vi "test_read-nmea-data2.vi"() -> ()   [LabVIEW 2019] (continued)
,57.96,250720,,,A,V*3D\n\t\n15:12:59.26\tF9P\t$GNVTG,57.96,T,,M,2.140,N,3.964,K,A*11\n\t\n15:12:59.28\tF9P\t$GNGGA,061301.00,3723.55169,N,12656.96549,E,1,12,0.94,42.1,M,18.5,M,,*78\n\t\n15:12:59.30\tF9P\t$GNGSA,A,3,12,06,19,05,17,09,04,02,,,,,1.64,0.94,1.34,1*08\n\t\n15:12:59.32\tF9P\t$GNGSA,A,3,85,70,71,84,,,,,,,,,1.64,0.94,1.34,2*0A\n\t\n15:12:59.34\tF9P\t$GNGSA,A,3,36,19,11,04,09,12,,,,,,,1.64,0.94,1.34,3*08\n\t\n15:12:59.36\tF9P\t$GNGSA,A,3,14,11,33,,,,,,,,,,1.64,0.94,1.34,4*09\n\t\n15:12:59.38\tF9P\t$GPGSV,3,1,09,02,55,319,21,04,18,043,25,05,37,247,27,06,64,049,31,1*66\n\t\n15:12:59.40\tF9P\t$GPGSV,3,2,09,09,45,074,34,12,23,276,25,17,33,154,30,19,52,157,31,1*6D\n\t\n15:12:59.42\tF9P\t$GPGSV,3,3,09,25,12,306,21,1*5F\n\t\n15:12:59.44\tF9P\t$GPGSV,3,1,09,02,55,319,,04,18,043,21,05,37,247,21,06,64,049,24,6*64\n\t\n15:12:59.46\tF9P\t$GPGSV,3,2,09,09,45,074,28,12,23,276,16,17,33,154,19,19,52,157,,6*6E\n\t\n15:12:59.48\tF9P\t$GPGSV,3,3,09,25,12,306,,6*5B\n\t\n15:12:59.50\tF9P\t$GLGSV,2,1,08,69,11,031,25,70,70,038,28,71,53,206,37,72,05,210,23,1*7A\n\t\n15:12:59.52\tF9P\t$GLGSV,2,2,08,77,01,326,,84,20,122,12,85,70,067,35,86,37,330,,1*7D\n\t\n15:12:59.54\tF9P\t$GLGSV,2,1,08,69,11,031,14,70,70,038,,71,53,206,26,72,05,210,,3*71\n\t\n15:12:59.56\tF9P\t$GLGSV,2,2,08,77,01,326,,84,20,122,19,85,70,067,29,86,37,330,,3*79\n\t\n15:12:59.58\tF9P\t$GAGSV,2,1,08,02,08,297,08,04,66,116,27,09,32,193,34,11,72,359,26,7*7B\n\t\n15:12:59.60\tF9P\t$GAGSV,2,2,08,12,40,103,33,19,26,045,22,25,09,249,,36,26,308,16,7*7F\n\t\n15:12:59.62\tF9P\t$GAGSV,2,1,08,02,08,297,,04,66,116,,09,32,193,32,11,72,359,,2*71\n\t\n15:12:59.64\tF9P\t$GAGSV,2,2,08,12,40,103,,19,26,045,,25,09,249,,36,26,308,,2*7D\n\t\n15:12:59.66\tF9P\t$GBGSV,1,1,04,11,49,132,24,14,87,114,27,28,,,20,33,61,220,35,1*4B\n\t\n15:12:59.68\tF9P\t$GBGSV,1,1,03,11,49,132,,14,87,114,27,33,61,220,,3*46\n\t\n15:12:59.70\tF9P\t$GNGLL,3723.55169,N,12656.96549,E,061301.00,A,A*78\n\t\n15:12:59.72\tF9P\t\t\n15:12:59.74\tF9P\t\t\n15:12:59.76\tF9P\t\t\n15:12:59.78\tF9P\t\t\n15:12:59.80\tF9P\t\t\n15:12:59.82\tF9P\t\t\n15:12:59.84\tF9P\t\t\n15:12:59.86\tF9P\t\t\n15:12:59.88\tF9P\t\t\n15:12:59.90\tF9P\t\t\n15:12:59.92\tF9P\t\t\n15:12:59.94\tF9P\t\t\n15:12:59.96\tF9P\t\t\n15:12:59.98\tF9P\t\t\n15:13:00.00\tF9P\t\t\n15:13:00.02\tF9P\t\t\n15:13:00.04\tF9P\t\t\n15:13:00.06\tF9P\t\t\n15:13:00.08\tF9P\t\t\n15:13:00.10\tF9P\t\t\n15:13:00.12\tF9P\t\t\n15:13:00.14\tF9P\t\t\n15:13:00.16\tF9P\t\t\n15:13:00.18\tF9P\t\t\n15:13:00.20\tF9P\t\t\n15:13:00.22\tF9P\t\t\n15:13:00.24\tF9P\t$GNRMC,061302.00,A,3723.55217,N,12656.96618,E,2.079,53.79,250720,,,A,V*3D\n\t\n15:13:00.26\tF9P\t$GNVTG,53.79,T,,M,2.079,N,3.851,K,A*18\n\t\n15:13:00.28\tF9P\t$GNGGA,061302.00,3723.55217,N,12656.96618,E,1,12,0.93,42.2,M,18.5,M,,*72\n\t\n15:13:00.30\tF9P\t$GNGSA,A,3,12,06,19,05,17,09,04,02,,,,,1.63,0.93,1.34,1*08\n\t\n15:13:00.32\tF9P\t$GNGSA,A,3,85,70,71,84,,,,,,,,,1.63,0.93,1.34,2*0A\n\t\n15:13:00.34\tF9P\t$GNGSA,A,3,36,19,11,04,09,12,,,,,,,1.63,0.93,1.34,3*08\n\t\n15:13:00.36\tF9P\t$GNGSA,A,3,14,11,33,,,,,,,,,,1.63,0.93,1.34,4*09\n\t\n15:13:00.38\tF9P\t$GPGSV,3,1,09,02,55,319,21,04,18,043,24,05,37,247,26,06,64,049,25,1*63\n\t\n15:13:00.40\tF9P\t$GPGSV,3,2,09,09,45,074,29,12,23,276,,17,33,154,33,19,52,157,29,1*6C\n\t\n15:13:00.42\tF9P\t$GPGSV,3,3,09,25,12,306,21,1*5F\n\t\n15:13:00.44\tF9P\t$GPGSV,3,1,09,02,55,319,,04,18,043,22,05,37,247,20,06,64,049,26,6*64\n\t\n15:13:00.46\tF9P\t$GPGSV,3,2,09,09,45,074,28,12,23,276,13,17,33,154,19,19,52,157,,6*6B\n\t\n15:13:00.48\tF9P\t$GPGSV,3,3,09,25,12,306,,6*5B\n\t\n15:13:00.50\tF9P\t$GLGSV,2,1,08,69,11,031,23,70,70,038,30,71,53,206,38,72,05,210,23,1*7A\n\t\n15:13:00.52\tF9P\t$GLGSV,2,2,08,77,01,326,,84,20,122,13,85,70,067,31,86,37,330,,1*78\n\t\n15:13:00.54\tF9P\t$GLGSV,2,1,08,69,11,031,15,70,70,038,,71,53,206,25,72,05,210,,3*73\n\t\n15:13:00.56\tF9P\t$GLGSV,2,2,08,77,01,326,,84,20,122,18,85,70,067,23,86,37,330,,3*72\n\t\n15:13:00.58\tF9P\t$GAGSV,2,1,08,02,08,297,12,04,66,116,28,09,32,193,33,11,72,359,31,7*7E\n\t\n15:13:00.60\tF9P\t$GAGSV,2,2,08,12,40,103,32,19,26,045,24,25,09,249,,36,26,308,15,7*7B\n\t\n15:13:00.62\tF9P\t$GAGSV,2,1,08,02,08,297,,04,66,116,,09,32,193,,11,72,359,,2*70\n\t\n15:13:00.64\tF9P\t$GAGSV,2,2,08,12,40,103,,19,26,045,,25,09,249,,36,26,308,,2*7D\n\t\n15:13:00.66\tF9P\t$GBGSV,1,1,04,11,49,132,30,14,87,114,28,28,,,21,33,61,220,27,1*43\n\t\n15:13:00.68\tF9P\t$GBGSV,1,1,03,11,49,132,,14,87,114,,33,61,220,,3*43\n\t\n15:13:00.70\tF9P\t$GNGLL,3723.55217,N,12656.96618,E,061302.00,A,A*76\n\t\n15:13:00.72\tF9P\t\t\n15:13:00.74\tF9P\t\t\n15:13:00.76\tF9P\t\t\n15:13:00.78\tF9P\t\t\n15:13:00.80\tF9P\t\t\n15:13:00.82\tF9P\t\t\n15:13:00.84\tF9P\t\t\n15:13:00.86\tF9P\t\t\n15:13:00.88\tF9P\t\t\n15:13:00.90\tF9P\t\t\n15:13:00.92\tF9P\t\t\n15:13:00.94\tF9P\t\t\n15:13:00.96\tF9P\t\t\n15:13:00.98\tF9P\t\t\n15:13:01.00\tF9P\t\t\n15:13:01.02\tF9P\t\t\n15:13:01.04\tF9P\t\t\n15:13:01.06\tF9P\t\t\n15:13:01.08\tF9P\t\t\n15:13:01.10\tF9P\t\t\n15:13:01.12\tF9P\t\t\n15:13:01.14\tF9P\t\t\n15:13:01.16\tF9P\t\t\n15:13:01.18\tF9P\t\t\n15:13:01.20\tF9P\t\t\n15:13:01.22\tF9P\t\t\n15:13:01.24\tF9P\t$GNRMC,061303.00,A,3723.55265,N,12656.96684,E,2.088,52.28,250720,,,A,V*37\n\t\n15:13:01.26\tF9P\t$GNVTG,52.28,T,,M,2.088,N,3.867,K,A*16\n\t\n15:13:01.28\tF9P\t$GNGGA,061303.00,3723.55265,N,12656.96684,E,1,12,0.93,42.2,M,18.5,M,,*73\n\t\n15:13:01.30\tF9P\t$GNGSA,A,3,06,19,05,17,09,04,02,,,,,,1.63,0.93,1.34,1*0B\n\t\n15:13:01.32\tF9P\t$GNGSA,A,3,85,70,71,84,,,,,,,,,1.63,0.93,1.34,2*0A\n\t\n15:13:01.34\tF9P\t$GNGSA,A,3,36,19,11,04,09,12,,,,,,,1.63,0.93,1.34,3*08\n\t\n15:13:01.36\tF9P\t$GNGSA,A,3,14,11,33,,,,,,,,,,1.63,0.93,1.34,4*09\n\t\n15:13:01.38\tF9P\t$GPGSV,3,1,09,02,55,319,21,04,18,043,25,05,37,247,35,06,64,049,34,1*60\n\t\n15:13:01.40\tF9P\t$GPGSV,3,2,09,09,45,074,33,12,23,276,23,17,33,154,29,19,52,157,34,1*61\n\t\n15:13:01.42\tF9P\t$GPGSV,3,3,09,25,12,306,21,1*5F\n\t\n15:13:01.44\tF9P\t$GPGSV,3,1,09,02,55,319,,04,18,043,21,05,37,247,21,06,64,049,25,6*65\n\t\n15:13:01.46\tF9P\t$GPGSV,3,2,09,09,45,074,26,12,23,276,,17,33,154,20,19,52,157,,6*6D\n\t\n15:13:01.48\tF9P\t$GPGSV,3,3,09,25,12,306,,6*5B\n\t\n15:13:01.50\tF9P\t$GLGSV,2,1,08,69,11,031,23,70,70,038,30,71,53,206,39,72,05,210,23,1*7B\n\t\n15:13:01.52\tF9P\t$GLGSV,2,2,08,77,01,326,,84,20,122,10,85,70,067,29,86,37,330,,1*72\n\t\n15:13:01.54\tF9P\t$GLGSV,2,1,08,69,11,031,17,70,70,038,,71,53,206,25,72,05,210,,3*71\n\t\n15:13:01.56\tF9P\t$GLGSV,2,2,08,77,01,326,,84,20,122,20,85,70,067,22,86,37,330,,3*78\n\t\n15:13:01.58\tF9P\t$GAGSV,2,1,08,02,08,297,12,04,66,116,28,09,32,193,34,11,72,359,31,7*79\n\t\n15:13:01.60\tF9P\t$GAGSV,2,2,08,12,40,103,28,19,26,045,24,25,09,249,,36,26,308,15,7*70\n\t\n15:13:01.62\tF9P\t$GAGSV,2,1,08,02,08,297,,04,66,116,,09,32,193,,11,72,359,,2*70\n\t\n15:13:01.64\tF9P\t$GAGSV,2,2,08,12,40,103,,19,26,045,,25,09,249,,36,26,308,,2*7D\n\t\n15:13:01.66\tF9P\t$GBGSV,1,1,04,11,49,132,29,14,87,114,32,28,,,20,33,61,220,32,1*45\n\t\n15:13:01.68\tF9P\t$GBGSV,1,1,03,11,49,132,,14,87,114,27,33,61,220,,3*46\n\t\n15:13:01.70\tF9P\t$GNGLL,3723.55265,N,12656.96684,E,061303.00,A,A*77\n\t\n15:13:01.72\tF9P\t\t\n15:13:01.74\tF9P\t\t\n15:13:01.76\tF9P\t\t\n15:13:01.78\tF9P\t\t\n15:13:01.80\tF9P\t\t\n15:13:01.82\tF9P\t\t\n15:13:01.84\tF9P\t\t\n15:13:01.86\tF9P\t\t\n15:13:01.88\tF9P\t\t\n15:13:01.90\tF9P\t\t\n15:13:01.92\tF9P\t\t\n15:13:01.94\tF9P\t\t\n15:13:01.96\tF9P\t\t\n15:13:01.98\tF9P\t\t\n15:13:02.00\tF9P\t\t\n15:13:02.02\tF9P\t\t\n15:13:02.04\tF9P\t\t\n15:13:02.06\tF9P\t\t\n15:13:02.08\tF9P\t\t\n15:13:02.10\tF9P\t\t\n15:13:02.12\tF9P\t\t\n15:13:02.14\tF9P\t\t\n15:13:02.16\tF9P\t\t\n15:13:02.18\tF9P\t\t\n15:13:02.20\tF9P\t\t\n15:13:02.22\tF9P\t\t\n15:13:02.24\tF9P\t$GNRMC,061304.00,A,3723.55321,N,12656.96735,E,1.731,50.68,250720,,,A,V*3A\n\t\n15:13:02.26\tF9P\t$GNVTG,50.68,T,,M,1.731,N,3.206,K,A*1B\n\t\n15:13:02.28\tF9P\t$GNGGA,061304.00,3723.55321,N,12656.96735,E,1,12,0.93,42.3,M,18.5,M,,*7F\n\t\n15:13:02.30\tF9P\t$GNGSA,A,3,06,19,05,17,09,04,02,,,,,,1.63,0.93,1.34,1*0B\n\t\n15:13:02.32\tF9P\t$GNGSA,A,3,85,70,71,84,,,,,,,,,1.63,0.93,1.34,2*0A\n\t\n15:13:02.34\tF9P\t$GNGSA,A,3,36,19,11,04,09,12,,,,,,,1.63,0.93,1.34,3*08\n\t\n15:13:02.36\tF9P\t$GNGSA,A,3,14,11,33,,,,,,,,,,1.63,0.93,1.34,4*09\n\t\n15:13:02.38\tF9P\t$GPGSV,3,1,09,02,55,319,22,04,18,043,26,05,37,247,30,06,64,049,25,1*65\n\t\n15:13:02.40\tF9P\t$GPGSV,3,2,09,09,45,074,31,12,23,276,23,17,33,154,28,19,52,157,30,1*66\n\t\n15:13:02.42\tF9P\t$GPGSV,3,3,09,25,12,306,20,1*5E\n\t\n15:13:02.44\tF9P\t$GPGSV,3,1,09,02,55,319,,04,18,043,19,05,37,247,22,06,64,049,25,6*6D\n\t\n15:13:02.46\tF9P\t$GPGSV,3,2,09,09,45,074,28,12,23,276,,17,33,154,20,19,52,157,,6*63\n\t\n15:13:02.48\tF9P\t$GPGSV,3,3,09,25,12,306,,6*5B\n\t\n15:13:02.50\tF9P\t$GLGSV,2,1,08,69,11,031,23,70,70,038,31,71,53,206,42,72,05,210,23,1*76\n\t\n15:13:02.52\tF9P\t$GLGSV,2,2,08,77,01,326,,84,20,122,15,85,70,067,34,86,37,330,,1*7B\n\t\n15:13:02.54\tF9P\t$GLGSV,2,1,08,69,11,031,16,70,70,038,,71,53,206,25,72,05,210,,3*70\n\t\n15:13:02.56\tF9P\t$GLGSV,2,2,08,77,01,326,,84,20,122,20,85,70,067,21,86,37,330,,3*7B\n\t\n15:13:02.58\tF9P\t$GAGSV,2,1,08,02,08,297,09,04,66,116,28,09,32,193,37,11,72,359,35,7*74\n\t\n15:13:02.60\tF9P\t$GAGSV,2,2,08,12,40,103,28,19,26,045,24,25,09,249,,36,26,308,16,7*73\n\t\n15:13:02.62\tF9P\t$GAGSV,2,1,08,02,08,297,,04,66,116,,09,32,193,,11,72,359,,2*70\n\t\n15:13:02.64\tF9P\t$GAGSV,2,2,08,12,40,103,,19,26,045,,25,09,249,,36,26,308,,2*7D\n\t\n15:13:02.66\tF9P\t$GBGSV,1,1,04,11,49,132,28,14,87,114,28,28,,,20,33,61,220,30,1*4D\n\t\n15:13:02.68\tF9P\t$GBGSV,1,1,03,11,49,132,,14,87,114,27,33,61,220,,3*46\n\t\n15:13:02.70\tF9P\t$GNGLL,3723.55321,N,12656.96735,E,061304.00,A,A*7A\n\t\n15:13:02.72\tF9P\t\t\n15:13:02.74\tF9P\t\t\n15:13:02.76\tF9P\t\t\n15:13:02.78\tF9P\t\t\n15:13:02.80\tF9P\t\t\n15:13:02.82\tF9P\t\t\n15:13:02.84\tF9P\t\t\n15:13:02.86\tF9P\t\t\n15:13:02.88\tF9P\t\t\n15:13:02.90\tF9P\t\t\n15:13:02.92\tF9P\t\t\n15:13:02.94\tF9P\t\t\n15:13:02.96\tF9P\t\t\n15:13:02.98\tF9P\t\t\n15:13:03.00\tF9P\t\t\n15:13:03.02\tF9P\t\t\n15:13:03.04\tF9P\t\t\n15:13:03.06\tF9P\t\t\n15:13:03.08\tF9P\t\t\n15:13:03.10\tF9P\t\t\n15:13:03.12\tF9P\t\t\n15:13:03.14\tF9P\t\t\n15:13:03.16\tF9P\t\t\n15:13:03.18\tF9P\t\t\n15:13:03.20\tF9P\t\t\n15:13:03.22\tF9P\t\t\n15:13:03.24\tF9P\t$GNRMC,061305.00,A,3723.55365,N,12656.96800,E,2.177,53.20,250720,,,A,V*3A\n\t\n15:13:03.26\tF9P\t$GNVTG,53.20,T,,M,2.177,N,4.032,K,A*11\n\t\n15:13:03.28\tF9P\t$GNGGA,061305.00,3723.55365,N,12656.96800,E,1,12,0.93,42.1,M,18.5,M,,*75\n\t\n15:13:03.30\tF9P\t$GNGSA,A,3,12,06,19,05,17,09,04,02,,,,,1.63,0.93,1.34,1*08\n\t\n15:13:03.32\tF9P\t$GNGSA,A,3,85,70,71,84,,,,,,,,,1.63,0.93,1.34,2*0A\n\t\n15:13:03.34\tF9P\t$GNGSA,A,3,36,19,11,04,09,12,,,,,,,1.63,0.93,1.34,3*08\n\t\n15:13:03.36\tF9P\t$GNGSA,A,3,14,11,33,,,,,,,,,,1.63,0.93,1.34,4*09\n\t\n15:13:03.38\tF9P\t$GPGSV,3,1,09,02,55,319,22,04,18,043,25,05,37,247,29,06,64,049,25,1*6E\n\t\n15:13:03.40\tF9P\t$GPGSV,3,2,09,09,45,074,28,12,23,276,22,17,33,154,29,19,52,157,30,1*6E\n\t\n15:13:03.42\tF9P\t$GPGSV,3,3,09,25,12,306,20,1*5E\n\t\n15:13:03.44\tF9P\t$GPGSV,3,1,09,02,55,319,,04,18,043,17,05,37,247,22,06,64,049,26,6*60\n\t\n15:13:03.46\tF9P\t$GPGSV,3,2,09,09,45,074,27,12,23,276,,17,33,154,20,19,52,157,,6*6C\n\t\n15:13:03.48\tF9P\t$GPGSV,3,3,09,25,12,306,,6*5B\n\t\n15:13:03.50\tF9P\t$GLGSV,2,1,08,69,11,031,30,70,70,038,26,71,53,206,42,72,05,210,23,1*72\n\t\n15:13:03.52\tF9P\t$GLGSV,2,2,08,77,01,326,,84,20,122,11,85,70,067,38,86,37,330,,1*73\n\t\n15:13:03.54\tF9P\t$GLGSV,2,1,08,69,11,031,18,70,70,038,,71,53,206,23,72,05,210,,3*78\n\t\n15:13:03.56\tF9P\t$GLGSV,2,2,08,77,01,326,,84,20,122,19,85,70,067,22,86,37,330,,3*72\n\t\n15:13:03.58\tF9P\t$GAGSV,2,1,08,02,08,297,08,04,66,116,28,09,32,193,36,11,72,359,29,7*79\n\t\n15:13:03.60\tF9P\t$GAGSV,2,2,08,12,40,103,28,19,26,045,25,25,09,249,,36,26,308,15,7*71\n\t\n15:13:03.62\tF9P\t$GAGSV,2,1,08,02,08,297,,04,66,116,,09,32,193,,11,72,359,,2*70\n\t\n15:13:03.64\tF9P\t$GAGSV,2,2,08,12,40,103,,19,26,045,,25,09,249,,36,26,308,,2*7D\n\t\n15:13:03.66\tF9P\t$GBGSV,1,1,04,11,49,132,29,14,87,114,29,28,,,19,33,61,220,33,1*44\n\t\n15:13:03.68\tF9P\t$GBGSV,1,1,03,11,49,132,,14,87,114,27,33,61,220,,3*46\n\t\n15:13:03.70\tF9P\t$GNGLL,3723.55365,N,12656.96800,E,061305.00,A,A*72\n\t\n15:13:03.72\tF9P\t\t\n15:13:03.74\tF9P\t\t\n15:13:03.76\tF9P\t\t\n15:13:03.78\tF9P\t\t\n15:13:03.80\tF9P\t\t\n15:13:03.82\tF9P\t\t\n15:13:03.84\tF9P\t\t\n15:13:03.86\tF9P\t\t\n15:13:03.88\tF9P\t\t\n15:13:03.90\tF9P\t\t\n15:13:03.92\tF9P\t\t\n15:13:03.94\tF9P\t\t\n15:13:03.96\tF9P\t\t\n15:13:03.98\tF9P\t\t\n15:13:04.00\tF9P\t\t\n15:13:04.02\tF9P\t\t\n15:13:04.04\tF9P\t\t\n15:13:04.06\tF9P\t\t\n15:13:04.08\tF9P\t\t\n15:13:04.10\tF9P\t\t\n15:13:04.12\tF9P\t\t\n15:13:04.14\tF9P\t\t\n15:13:04.16\tF9P\t\t\n15:13:04.18\tF9P\t\t\n15:13:04.20\tF9P\t\t\n15:13:04.22\tF9P\t\t\n15:13:04.24\tF9P\t$GNRMC,061306.00,A,3723.55373,N,12656.96887,E,2.176,59.83,250720,,,A,V*33\n\t\n15:13:04.26\tF9P\t$GNVTG,59.83,T,,M,2.176,N,4.029,K,A*19\n\t\n15:13:04.28\tF9P\t$GNGGA,061306.00,3723.55373,N,12656.96887,E,1,12,0.93,43.8,M,18.5,M,,*76\n\t\n15:13:04.30\tF9P\t$GNGSA,A,3,12,06,19,05,17,09,04,02,,,,,1.63,0.93,1.34,1*08\n\t\n15:13:04.32\tF9P\t$GNGSA,A,3,85,70,71,84,,,,,,,,,1.63,0.93,1.34,2*0A\n\t\n15:13:04.34\tF9P\t$GNGSA,A,3,36,19,11,04,09,12,,,,,,,1.63,0.93,1.34,3*08\n\t\n15:13:04.36\tF9P\t$GNGSA,A,3,14,11,33,,,,,,,,,,1.63,0.93,1.34,4*09\n\t\n15:13:04.38\tF9P\t$GPGSV,3,1,09,02,55,319,22,04,18,043,25,05,37,247,33,06,64,049,31,1*60\n\t\n15:13:04.40\tF9P\t$GPGSV,3,2,09,09,45,074,29,12,23,276,21,17,33,154,29,19,52,157,30,1*6C\n\t\n15:13:04.42\tF9P\t$GPGSV,3,3,09,25,12,306,20,1*5E\n\t\n15:13:04.44\tF9P\t$GPGSV,3,1,09,02,55,319,,04,18,043,17,05,37,247,21,06,64,049,24,6*61\n\t\n15:13:04.46\tF9P\t$GPGSV,3,2,09,09,45,074,28,12,23,276,,17,33,154,20,19,52,157,,6*63\n\t\n15:13:04.48\tF9P\t$GPGSV,3,3,09,25,12,306,,6*5B\n\t\n15:13:04.50\tF9P\t$GLGSV,2,1,08,69,11,031,25,70,70,038,26,71,53,206,41,72,05,210,21,1*77\n\t\n15:13:04.52\tF9P\t$GLGSV,2,2,08,77,01,325,,84,20,122,12,85,70,067,32,86,37,330,,1*79\n\t\n15:13:04.54\tF9P\t$GLGSV,2,1,08,69,11,031,16,70,70,038,,71,53,206,24,72,05,210,,3*71\n\t\n15:13:04.56\tF9P\t$GLGSV,2,2,08,77,01,325,,84,20,122,19,85,70,067,23,86,37,330,,3*70\n\t\n15:13:04.58\tF9P\t$GAGSV,2,1,08,02,08,297,10,04,66,116,28,09,32,193,38,11,72,359,32,7*74\n\t\n15:13:04.60\tF9P\t$GAGSV,2,2,08,12,40,103,29,19,26,045,25,25,09,249,,36,26,308,14,7*71\n\t\n15:13:04.62\tF9P\t$GAGSV,2,1,08,02,08,297,,04,66,116,,09,32,193,,11,72,359,,2*70\n\t\n15:13:04.64\tF9P\t$GAGSV,2,2,08,12,40,103,,19,26,045,,25,09,249,,36,26,308,,2*7D\n\t\n15:13:04.66\tF9P\t$GBGSV,1,1,04,11,49,132,30,14,87,114,22,28,,,19,33,61,220,32,1*46\n\t\n15:13:04.68\tF9P\t$GBGSV,1,1,03,11,49,132,,14,87,114,26,33,61,220,,3*47\n\t\n15:13:04.70\tF9P\t$GNGLL,3723.55373,N,12656.96887,E,061306.00,A,A*79\n\t\n15:13:04.72\tF9P\t\t\n15:13:04.74\tF9P\t\t\n15:13:04.76\tF9P\t\t\n15:13:04.78\tF9P\t\t\n15:13:04.80\tF9P\t\t\n15:13:04.82\tF9P\t\t\n15:13:04.84\tF9P\t\t\n15:13:04.86\tF9P\t\t\n15:13:04.88\tF9P\t\t\n15:13:04.90\tF9P\t\t\n15:13:04.92\tF9P\t\t\n15:13:04.94\tF9P\t\t\n15:13:04.96\tF9P\t\t\n15:13:04.98\tF9P\t\t\n15:13:05.00\tF9P\t\t\n15:13:05.02\tF9P\t\t\n15:13:05.04\tF9P\t\t\n15:13:05.06\tF9P\t\t\n15:13:05.08\tF9P\t\t\n15:13:05.10\tF9P\t\t\n15:13:05.12\tF9P\t\t\n15:13:05.14\tF9P\t\t\n15:13:05.16\tF9P\t\t\n15:13:05.18\tF9P\t\t\n15:13:05.20\tF9P\t\t\n15:13:05.22\tF9P\t\t\n15:13:05.24\tF9P\t$GNRMC,061307.00,A,3723.55392,N,12656.96968,E,2.056,68.99,250720,,,A,V*37\n\t\n15:13:05.26\tF9P\t$GNVTG,68.99,T,,M,2.056,N,3.808,K,A*1F\n\t\n15:13:05.28\tF9P\t$GNGGA,061307.00,3723.55392,N,12656.96968,E,1,12,0.93,43.6,M,18.5,M,,*76\n\t\n15:13:05.30\tF9P\t$GNGSA,A,3,12,06,19,05,17,09,04,02,,,,,1.63,0.93,1.34,1*08\n\t\n15:13:05.32\tF9P\t$GNGSA,A,3,85,70,71,84,,,,,,,,,1.63,0.93,1.34,2*0A\n\t\n15:13:05.34\tF9P\t$GNGSA,A,3,36,19,11,04,09,12,,,,,,,1.63,0.93,1.34,3*08\n\t\n15:13:05.36\tF9P\t$GNGSA,A,3,14,11,33,,,,,,,,,,1.63,0.93,1.34,4*09\n\t\n15:13:05.38\tF9P\t$GPGSV,3,1,09,02,55,319,22,04,18,043,25,05,37,247,35,06,64,049,36,1*61\n\t\n15:13:05.40\tF9P\t$GPGSV,3,2,09,09,45,074,29,12,23,276,22,17,33,154,30,19,52,157,34,1*63\n\t\n15:13:05.42\tF9P\t$GPGSV,3,3,09,25,12,306,20,1*5E\n\t\n15:13:05.44\tF9P\t$GPGSV,3,1,09,02,55,319,,04,18,043,17,05,37,247,20,06,64,049,25,6*61\n\t\n15:13:05.46\tF9P\t$GPGSV,3,2,09,09,45,074,28,12,23,276,,17,33,154,22,19,52,157,,6*61\n\t\n15:13:05.48\tF9P\t$GPGSV,3,3,09,25,12,306,,6*5B\n\t\n15:13:05.50\tF9P\t$GLGSV,2,1,08,69,11,031,25,70,70,038,26,71,53,206,35,72,05,210,20,1*75\n\t\n15:13:05.52\tF9P\t$GLGSV,2,2,08,77,01,325,,84,20,122,13,85,70,067,29,86,37,330,,1*72\n\t\n15:13:05.54\tF9P\t$GLGSV,2,1,08,69,11,031,18,70,70,038,,71,53,206,31,72,05,210,,3*7B\n\t\n15:13:05.56\tF9P\t$GLGSV,2,2,08,77,01,325,,84,20,122,19,85,70,067,25,86,37,330,,3*76\n\t\n15:13:05.58\tF9P\t$GAGSV,2,1,08,02,08,297,12,04,66,116,33,09,32,193,33,11,72,359,27,7*73\n\t\n15:13:05.60\tF9P\t$GAGSV,2,2,08,12,40,103,30,19,26,045,22,25,09,249,,36,26,308,13,7*79\n\t\n15:13:05.62\tF9P\t$GAGSV,2,1,08,02,08,297,,04,66,116,,09,32,193,,11,72,359,,2*70\n\t\n15:13:05.64\tF9P\t$GAGSV,2,2,08,12,40,103,,19,26,045,,25,09,249,,36,26,308,,2*7D\n\t\n15:13:05.66\tF9P\t$GBGSV,1,1,04,11,49,132,33,14,87,114,29,28,,,20,33,61,220,34,1*42\n\t\n15:13:05.68\tF9P\t$GBGSV,1,1,03,11,49,132,,14,87,114,,33,61,220,,3*43\n\t\n15:13:05.70\tF9P\t$GNGLL,3723.55392,N,12656.96968,E,061307.00,A,A*77\n\t\n15:13:05.72\tF9P\t\t\n15:13:05.74\tF9P\t\t\n15:13:05.76\tF9P\t\t\n15:13:05.78\tF9P\t\t\n15:13:05.80\tF9P\t\t\n15:13:05.82\tF9P\t\t\n15:13:05.84\tF9P\t\t\n15:13:05.86\tF9P\t\t\n15:13:05.88\tF9P\t\t\n15:13:05.90\tF9P\t\t\n15:13:05.92\tF9P\t\t\n15:13:05.94\tF9P\t\t\n15:13:05.96\tF9P\t\t\n15:13:05.98\tF9P\t\t\n15:13:06.00\tF9P\t\t\n15:13:06.02\tF9P\t\t\n15:13:06.04\tF9P\t\t\n15:13:06.06\tF9P\t\t\n15:13:06.08\tF9P\t\t\n15:13:06.10\tF9P\t\t\n15:13:06.12\tF9P\t\t\n15:13:06.14\tF9P\t\t\n15:13:06.16\tF9P\t\t\n15:13:06.18\tF9P\t\t\n15:13:06.20\tF9P\t\t\n15:13:06.22\tF9P\t\t\n15:13:06.24\tF9P\t$GNRMC,061308.00,A,3723.55442,N,12656.97048,E,2.371,69.27,250720,,,A,V*3A\n\t\n15:13:06.26\tF9P\t$GNVTG,69.27,T,,M,2.371,N,4.391,K,A*11\n\t\n15:13:06.28\tF9P\t$GNGGA,061308.00,3723.55442,N,12656.97048,E,1,12,0.94,42.4,M,18.5,M,,*7D\n\t\n15:13:06.30\tF9P\t$GNGSA,A,3,12,06,19,05,17,09,04,02,,,,,1.65,0.94,1.35,1*08\n\t\n15:13:06.32\tF9P\t$GNGSA,A,3,85,71,84,,,,,,,,,,1.65,0.94,1.35,2*0D\n\t\n15:13:06.34\tF9P\t$GNGSA,A,3,36,19,11,04,09,12,,,,,,,1.65,0.94,1.35,3*08\n\t\n15:13:06.36\tF9P\t$GNGSA,A,3,14,11,33,,,,,,,,,,1.65,0.94,1.35,4*09\n\t\n15:13:06.38\tF9P\t$GPGSV,3,1,09,02,55,319,21,04,18,043,25,05,37,247,37,06,64,049,29,1*6E\n\t\n15:13:06.40\tF9P\t$GPGSV,3,2,09,09,45,074,30,12,23,276,22,17,33,154,34,19,52,157,28,1*62\n\t\n15:13:06.42\tF9P\t$GPGSV,3,3,09,25,12,306,20,1*5E\n\t\n15:13:06.44\tF9P\t$GPGSV,3,1,09,02,55,319,,04,18,043,16,05,37,247,19,06,64,049,26,6*69\n\t\n15:13:06.46\tF9P\t$GPGSV,3,2,09,09,45,074,36,12,23,276,,17,33,154,21,19,52,157,,6*6D\n\t\n15:13:06.48\tF9P\t$GPGSV,3,3,09,25,12,306,,6*5B\n\t\n15:13:06.50\tF9P\t$GLGSV,2,1,08,69,11,031,25,70,70,038,23,71,53,206,30,72,05,210,18,1*7E\n\t\n15:13:06.52\tF9P\t$GLGSV,2,2,08,77,01,325,,84,20,122,13,85,70,067,33,86,37,330,,1*79\n\t\n15:13:06.54\tF9P\t$GLGSV,2,1,08,69,11,031,20,70,70,038,,71,53,206,26,72,05,210,,3*76\n\t\n15:13:06.56\tF9P\t$GLGSV,2,2,08,77,01,325,,84,20,122,20,85,70,067,30,86,37,330,,3*78\n\t\n15:13:06.58\tF9P\t$GAGSV,2,1,08,02,08,297,08,04,66,116,33,09,32,193,27,11,72,359,27,7*7D\n\t\n15:13:06.60\tF9P\t$GAGSV,2,2,08,12,40,103,29,19,26,045,22,25,09,249,,36,26,308,12,7*70\n\t\n15:13:06.62\tF9P\t$GAGSV,2,1,08,02,08,297,,04,66,116,,09,32,193,,11,72,359,,2*70\n\t\n15:13:06.64\tF9P\t$GAGSV,2,2,08,12,40,103,,19,26,045,,25,09,249,,36,26,308,,2*7D\n\t\n15:13:06.66\tF9P\t$GBGSV,1,1,04,11,49,132,27,14,87,114,29,28,,,21,33,61,220,36,1*44\n\t\n15:13:06.68\tF9P\t$GBGSV,1,1,03,11,49,132,30,14,87,114,,33,61,220,,3*40\n\t\n15:13:06.70\tF9P\t$GNGLL,3723.55442,N,12656.97048,E,061308.00,A,A*78\n\t\n15:13:06.72\tF9P\t\t\n15:13:06.74\tF9P\t\t\n15:13:06.76\tF9P\t\t
